vi "Disconnect.vi"(8 "error in":errorcluster, 11 "CanHandleIn":T1) -> (0 "error out":errorcluster)   [LabVIEW 2011, in "Konvolucio MCAN120803.lvlib"]
doc: "Disconnect and freeing resources."
uses:
  <instrlib>/Konvolucio MCAN120803/Konvolucio MCAN120803.lvlib
  <instrlib>/Konvolucio MCAN120803/Types/CanHandleType.ctl
  C:/Program Files/National Instruments/LabVIEW 2011/instr.lib/Konvolucio MCAN120803/Private/Konvolucio.MCAN120803.API.dll
  Private/Konvolucio.MCAN120803.API.dll
  <instrlib>/Konvolucio MCAN120803/Public/Attributes/AttrGetIsConnected.vi
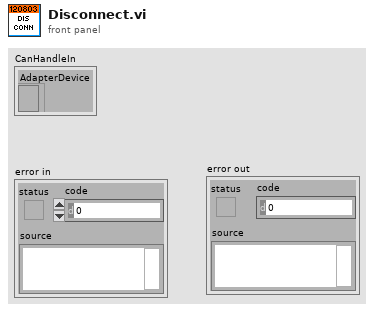
[diagram p1: front panel]
types:
  T1 = typedef "Konvolucio MCAN120803.lvlib/CanHandleType.ctl" = cluster{"AdapterDevice":refnum<k24>}
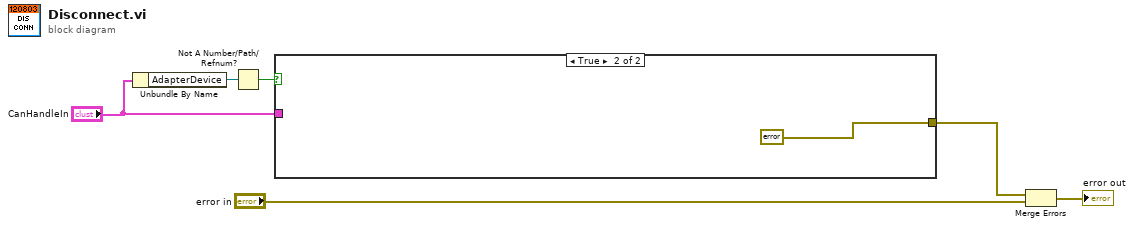
[diagram p0: block diagram]
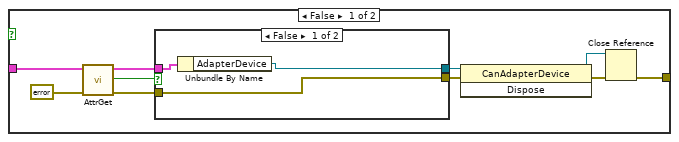
[diagram p2: hidden frame]
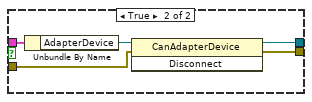
[diagram p3: hidden frame]
diagram:
  n1 = Unbundle By Name("CanHandleIn") -> ("AdapterDevice"=w3:refnum<k24>)
  n2 = Not A Number/Path/Refnum?(number/path/refnum=w3) -> (NaN/Path/Refnum?=w1:bool)
  n3 = case shown="True" w1 {
    tunnel: "CanHandleIn" -> [w12 _]
    tunnel: [w9 errorcluster {"status"=FALSE, "code"=0, "source"=""} ("error out")] -> w2
    frame False {
      n4 = call-poly <instrlib>:"AttrGet.vi"("error in"=errorcluster {"status"=FALSE, "code"=0, "source"=""} ("error in (no error)"), "CanHandleIn"=w12) -> ("error out"=w16:errorcluster, "State"=w13:bool, "CanHandleOut"=w15:T1)  [unwired: 7 in]
      n5 = case shown="False" w13 {
        tunnel: [w19 w21] -> w11
        tunnel: w16 -> [w19 w22]
        tunnel: w15 -> [w18 w24]
        tunnel: [w17 w20] -> w10
        frame False {
          n6 = Unbundle By Name(w18) -> ("AdapterDevice"=w17:refnum<k24>)
        }
        frame True {
          n7 = Unbundle By Name(w24) -> ("AdapterDevice"=w23:refnum<k24>)
          n8 = invoke class="CanAdapterDevice" method="Disconnect"(reference=w23, error in=w22) -> (reference out=w20:refnum<k24>, error out=w21:errorcluster)  [unwired: 1 in, 1 out]
        }
      }
      n9 = invoke class="CanAdapterDevice" method="Dispose"(reference=w10, error in=w11) -> (reference out=w7:refnum<k24>, error out=w8:errorcluster)  [unwired: 1 in, 1 out]
      n10 = Close Reference(reference=w7, error in (no error)=w8) -> (error out=w9:errorcluster)
    }
    frame True {
    }
  }
  n11 = Merge Errors(w2, "error in") -> (→"error out":errorcluster)
